vi "Doc_Builder_Set_Font.vi"(11 "NI_report in":refnum<class "NI_report.lvclass">) -> (3 "NI_report out":refnum<class "NI_report.lvclass">)   [LabVIEW 2019]
uses:
  <vilib>/Utility/NIReport.llb/NI_report.lvclass
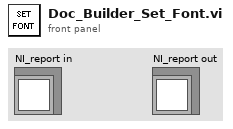
[diagram p1: front panel]
types:
  T1 = cluster{"Charset (-1)":i16, "Weight (-1)":i16, "Name":string, "Size":string}
  T2 = cluster{"Italic":enum16{"Italic Unchanged", "Italic On", "Italic Off"}, "Strike Through":enum16{"Strike Through Unchanged", "Strike Through On", "Strike Through Off"}, "Underline":enum16{"Underline Unchanged", "Underline On", "Underline Off"}, "Bold":enum16{"Bold Unchanged", "Bold On", "Bold Off"}}
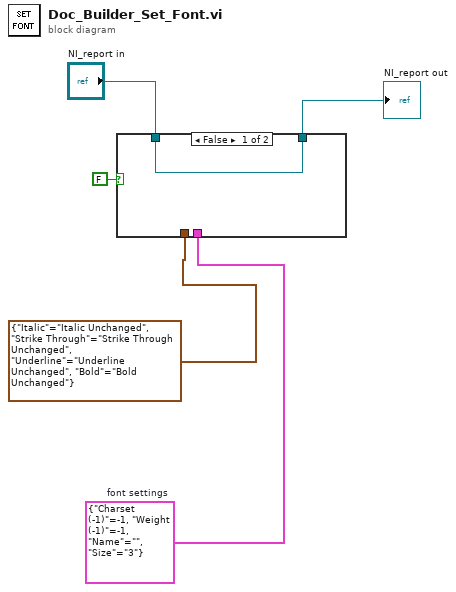
[diagram p0: block diagram]
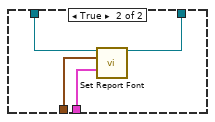
[diagram p2: hidden frame]
diagram:
  w2 = T1 {"Charset (-1)"=-1, "Weight (-1)"=-1, "Name"="", "Size"="3"}  # font settings
  n1 = case shown="False" FALSE {
    tunnel: [w6 w10] -> w5
    tunnel: "NI_report in" -> [w6 w9]
    tunnel: T2 {"Italic"=enum."Italic Unchanged", "Strike Through"=enum."Strike Through Unchanged", "Underline"=enum."Underline Unchanged", "Bold"=enum."Bold Unchanged"} ("text options") -> [_ w8]
    tunnel: w2 -> [_ w7]
    frame False {
    }
    frame True {
      n2 = call-dynamic "Set Report Font.vi"("report in"=w9, "text options"=w8, "font settings"=w7) -> ("report out"=w10:refnum<class "NI_report.lvclass">)  [unwired: 10 in, 2 out]
    }
  }
  "NI_report out" <- w5
